vi "CLD 16 Add process.vi"(8 "error in (no error)":errorcluster, 11 "Cluster in":T1 {"Status Panel"."Process Value" format="%#.3g"; "Control Panel Array"."Tons of Peanuts" scale=0.0..10.0}) -> (0 "error out":errorcluster, 3 "Cluster out":T1 {"Status Panel"."Process Value" format="%#.3g"; "Control Panel Array"."Tons of Peanuts" scale=0.0..10.0})   [LabVIEW 2019]
doc: "CLD 16 exercise\n\nThis SubVI simulates the processing requirements and is called when the Use button is pressed. It includes a short delay during which time the Use button is disabled."
uses:
  CLD 16 Data Cluster.ctl
  CLD 16 Control Panel.ctl
  CLD 16 Status Panel.ctl
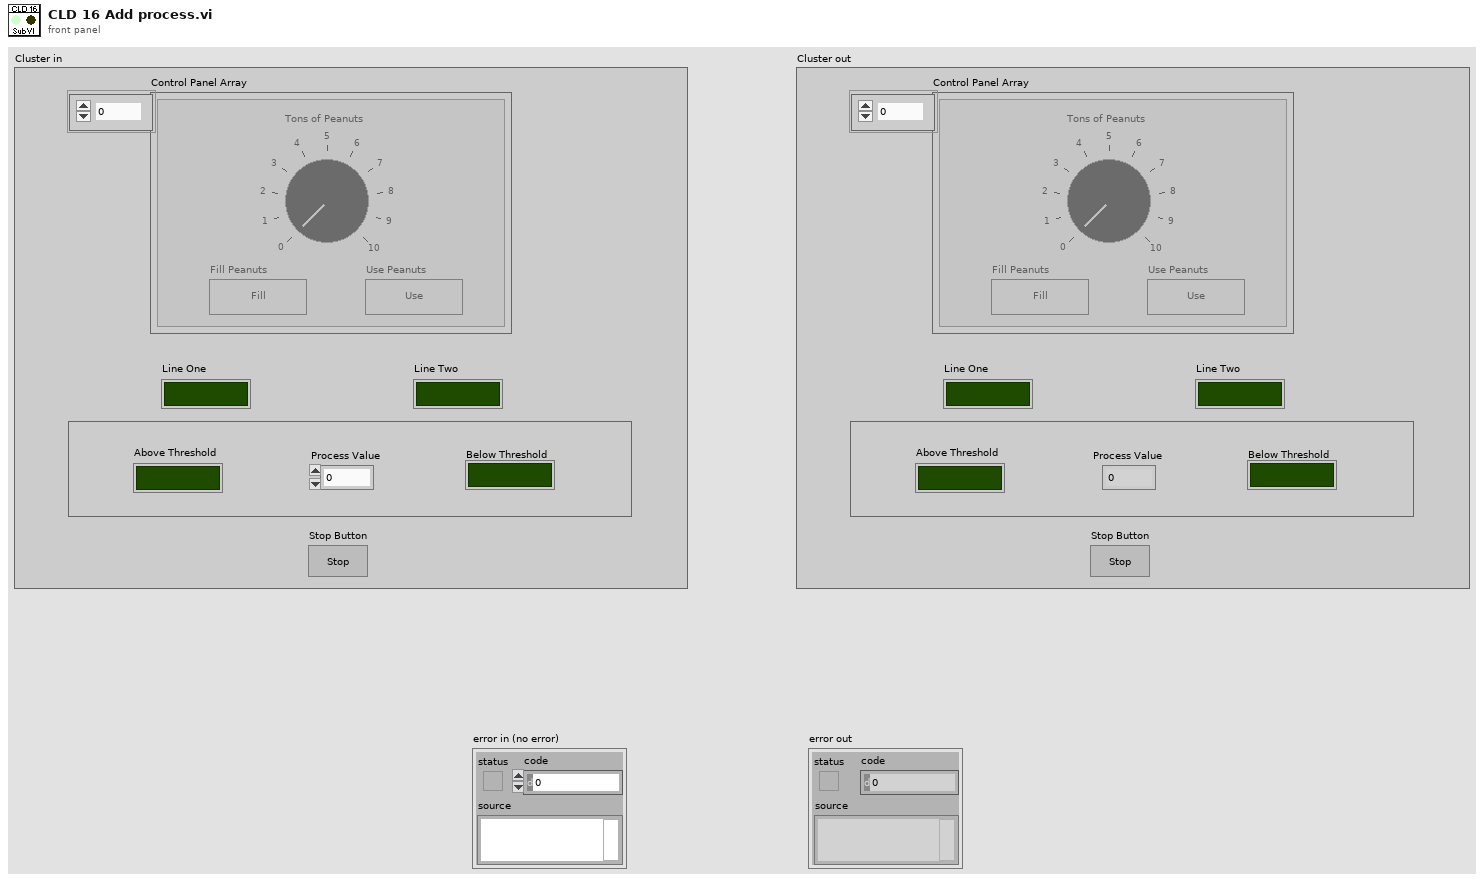
[diagram p1: front panel]
types:
  T1 = typedef "CLD 16 Data Cluster.ctl" = cluster{"Control Panel Array":T2[], "Status Panel":T3, "Line One":bool, "Line Two":bool, "Stop Button":bool}
  T2 = typedef "CLD 16 Control Panel.ctl" = cluster{"Tons of Peanuts":i8, "Fill Peanuts":bool, "Use Peanuts":bool}
  T3 = typedef "CLD 16 Status Panel.ctl" = cluster{"Above Threshold":bool, "Below Threshold":bool, "Process Value":dbl}
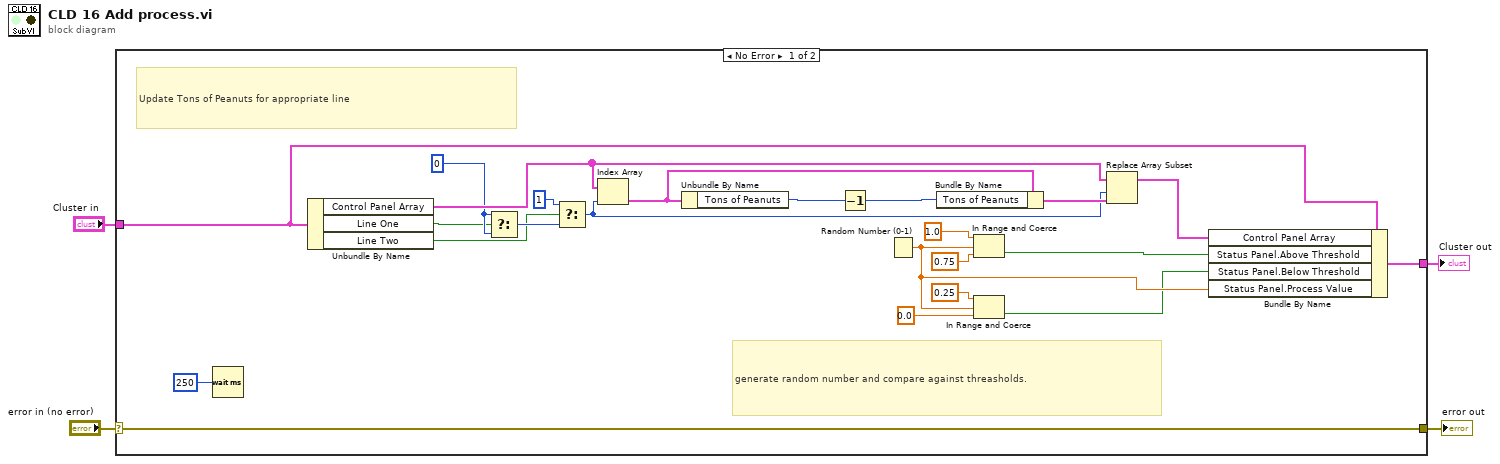
[diagram p0: block diagram]
diagram:
  n1 = case shown="No Error" "error in (no error)" {
    selector: "error in (no error)" -> [w6 w28]
    tunnel: [w27 w29] -> w4
    tunnel: "Cluster in" -> [w25 w29]
    tunnel: [w6 w28] -> w1
    frame No Error {
      w18 = 0
      # "Update Tons of Peanuts for appropriate line"
      # "generate random number and compare against threasholds."
      n2 = Wait (ms)(milliseconds to wait=u32 250) -> ()  [unwired: 1 out]
      n3 = Unbundle By Name(w25) -> ("Control Panel Array"=w22:T2[], "Line One"=w14:bool, "Line Two"=w15:bool)
      n4 = Select(t=w18, s=w14, f=w18) -> (s? t:f=w16:i32)
      n5 = Select(t=1, s=w15, f=w16) -> (s? t:f=w23:i32)
      n6 = Index Array(array=w22, index=w23) -> (element=w19:T2)
      n7 = Unbundle By Name(w19) -> ("Tons of Peanuts"=w20:i8)
      n8 = Decrement(x=w20) -> (x-1=w21:i8)
      n9 = Random Number (0-1)() -> (number: 0 to 1=w9:dbl)
      n10 = Bundle By Name(cluster=w19, "Tons of Peanuts"=w21) -> (w24:T2)
      n11 = In Range and Coerce(upper limit=1.0, x=w9, lower limit=0.75) -> (In Range?=w8:bool)  [unwired: 1 out]
      n12 = In Range and Coerce(upper limit=0.25, x=w9, lower limit=0.0) -> (In Range?=w7:bool)  [unwired: 1 out]
      n13 = Replace Array Subset(array=w22, new element=w24, index=w23) -> (w26:T2[])
      n14 = Bundle By Name(cluster=w25, "Control Panel Array"=w26, "Status Panel.Above Threshold"=w8, "Status Panel.Below Threshold"=w7, "Status Panel.Process Value"=w9) -> (w27:T1)
    }
    frame Error {
    }
  }
  "Cluster out" <- w4
  "error out" <- w1
